vi "FirstPrac1.vi"() -> ()   [LabVIEW 2018]
panel:
  out "Waveform Graph 3":cluster{dbl, dbl, dbl[]}(graph)
  out "Waveform Graph":cluster{dbl, dbl, dbl[]}(graph)
  in  "Stop":bool
  out "Waveform Chart":dbl(graph)
  out "String controller":string
  in  "String":string
  out "C * ( A + B )":dbl
  in  "Value C":dbl
  out "Counter":dbl
  in  "stop":bool
  out "A + B":dbl
  in  "Value B":dbl
  in  "Value A":dbl
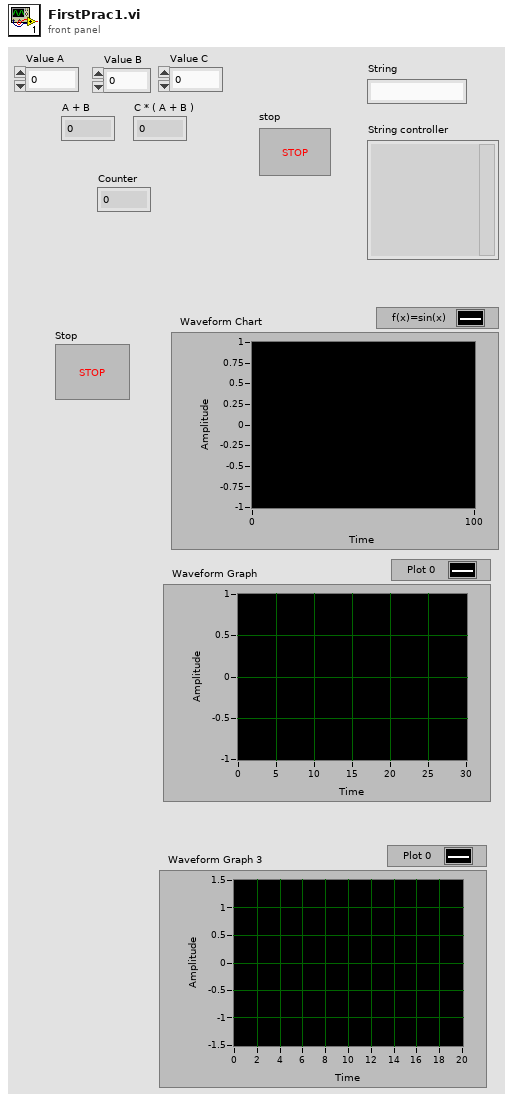
[diagram p1: front panel]
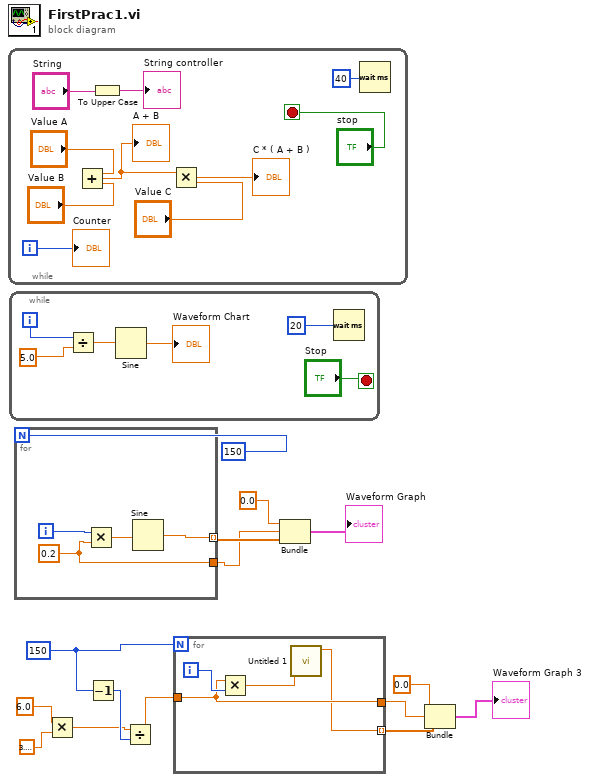
[diagram p0: block diagram]
diagram:
  w7 = 150
  n1 = while {
    i -> [w22]
    stop <- "stop" stop-if-true
    n2 = Add(x="Value A", y="Value B") -> (x+y=w21:dbl)
    "A + B" <- w21
    n3 = To Upper Case(1:"String") -> (0:→"String controller":string)
    n4 = Multiply(x=w21, y="Value C") -> (x*y=→"C * ( A + B )":dbl)
    n5 = Wait (ms)(milliseconds to wait=u32 40) -> ()  [unwired: 1 out]
    "Counter" <- w22
  }
  n6 = while {
    i -> [w27]
    stop <- "Stop" stop-if-true
    n7 = Divide(x=w27, y=5.0) -> (x/y=w29:dbl)
    n8 = Sine(x=w29) -> (sin(x)=→"Waveform Chart":dbl)
    n9 = Wait (ms)(milliseconds to wait=20) -> ()  [unwired: 1 out]
  }
  n10 = for {
    N: 150 -> [_]
    tunnel: [w35] -> w13 mode=indexing
    tunnel: [w32] -> w11
    i -> [w33]
    w32 = 0.2
    n11 = Multiply(x=w33, y=w32) -> (x*y=w34:dbl)
    n12 = Sine(x=w34) -> (sin(x)=w35:dbl)
  }
  n13 = Multiply(x=6.0, y=3.141592653589793) -> (x*y=w3:dbl)
  n14 = Decrement(x=w7) -> (x-1=w4:i32)
  n15 = Divide(x=w3, y=w4) -> (x/y=w2:dbl)
  n16 = for {
    N: w7 -> [_]
    tunnel: [w36] -> w8 mode=indexing
    tunnel: [w38] -> w9
    tunnel: w2 -> [w38]
    i -> [w39]
    n17 = Multiply(x=w38, y=w39) -> (x*y=w37:dbl)
    n18 = call "Untitled 1.vi"("x"=w37) -> ("sin sum(x)"=w36:dbl)  [unwired: 10 in]
  }
  n19 = Bundle(0.0, w11, w13) -> (→"Waveform Graph":cluster{dbl, dbl, dbl[]})  [unwired: 1 in]
  n20 = Bundle(0.0, w9, w8) -> (→"Waveform Graph 3":cluster{dbl, dbl, dbl[]})  [unwired: 1 in]
